vi "Test Lockin API.vi"() -> ()   [LabVIEW 2019]
uses:
  src/Instrument.Lockin/Instrument.Lockin.lvclass
  C:/Program Files (x86)/National Instruments/LabVIEW 2019/user.lib/LevyLab/Levylab Instruments/SMOs/Instrument/Instrument.lvclass
  src/Instrument.Lockinl.UI/Typedefs/Device Configuration--Cluster.ctl
  src/Lockin.DAQ/Typedefs/446xAO-enum.ctl
  src/Lockin.DAQ/Typedefs/446xAI-enum.ctl
  src/Lockin.DAQ/Typedefs/AI.coupling-enum.ctl
  <vilib>/addons/_JKI Toolkits/Caraya/classes/Test Suite/Define Test Suite (Default).vi
  <vilib>/addons/_JKI Toolkits/Caraya/classes/Test Suite/Test Suite.lvclass
  src/Lockin.DAQ/Lockin.DAQ.lvclass
  src/Instrument.Lockinl.UI/Instrument.Lockin.UI.lvclass
  <userlib>/LevyLab/Levylab Instruments/SMOs/Instrument/Instrument.lvclass
  C:/Program Files (x86)/National Instruments/LabVIEW 2019/vi.lib/JKI/JKI SMO/SMO/SMO.lvclass
panel:
  out "Instrument.Lockin out":refnum<class "Instrument.Lockin.lvclass">
  in  "Instrument.Lockin in":refnum<class "Instrument.Lockin.lvclass">
  # "NOTE:\nBefore running make sure that \"Same f\" = FALSE"
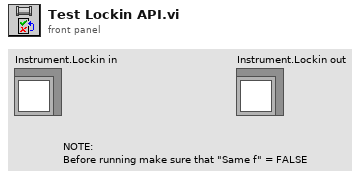
[diagram p1: front panel]
types:
  T1 = typedef "Instrument.Lockin.UI.lvclass/Device Configuration--Cluster.ctl" = cluster{"Device":string, "AO.Ch":string, "AO.Range":T2, "AI.Ch":string, "AI.Range":T3, "AI.Coupling":T4}
  T2 = typedef "Lockin.DAQ.lvclass/446xAO-enum.ctl" = enum16{"±0.1", "±1.0", "±10.0"}
  T3 = typedef "Lockin.DAQ.lvclass/446xAI-enum.ctl" = enum16{"±0.316", "±1.00", "±3.16", "±10.0", "±31.6", "±42.4"}
  T4 = typedef "Lockin.DAQ.lvclass/AI.coupling-enum.ctl" = u16
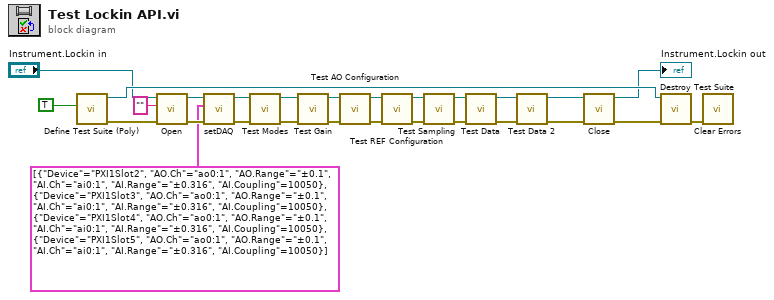
[diagram p0: block diagram]
diagram:
  n1 = call-poly <vilib>:"Define Test Suite (Poly).vi"("Interactive"=TRUE) -> ("error out"=w13:errorcluster, "Test Suite"=w22:refnum<class "Test Suite.lvclass">)  [unwired: 9 in]
  n2 = call <userlib>:"Open.vi"("error in (no error)"=w13, "address"="" ("Address"), "Instrument in"="Instrument.Lockin in") -> ("error out"=w9:errorcluster, "Instrument out"=w8:refnum<class "Instrument.Lockin.lvclass">)  [unwired: 7 in]
  n3 = call "setDAQ.vi"("error in (no error)"=w9, "setDAQ"=T1[] [{"Device"="PXI1Slot2", "AO.Ch"="ao0:1", "AO.Range"=enum."±0.1", "AI.Ch"="ai0:1", "AI.Range"=enum."±0.316", "AI.Coupling"=10050}, {"Device"="PXI1Slot3", "AO.Ch"="ao0:1", "AO.Range"=enum."±0.1", "AI.Ch"="ai0:1", "AI.Range"=enum."±0.316", "AI.Coupling"=10050}, {"Device"="PXI1Slot4", "AO.Ch"="ao0:1", "AO.Range"=enum."±0.1", "AI.Ch"="ai0:1", "AI.Range"=enum."±0.316", "AI.Coupling"=10050}, {"Device"="PXI1Slot5", "AO.Ch"="ao0:1", "AO.Range"=enum."±0.1", "AI.Ch"="ai0:1", "AI.Range"=enum."±0.316", "AI.Coupling"=10050}], "Instrument.Lockin in"=w8) -> ("error out"=w6:errorcluster, "Instrument.Lockin out"=w7:refnum<class "Instrument.Lockin.lvclass">)  [unwired: 7 in]
  n4 = call "Test Modes.vi"("error in (no error)"=w6, "Instrument.Lockin in"=w7) -> ("error out"=w21:errorcluster, "Instrument.Lockin out"=w27:refnum<class "Instrument.Lockin.lvclass">)  [unwired: 8 in]
  n5 = call "Test Gain.vi"("error in (no error)"=w21, "Instrument.Lockin in"=w27) -> ("error out"=w20:errorcluster, "Instrument.Lockin out"=w26:refnum<class "Instrument.Lockin.lvclass">)  [unwired: 8 in]
  n6 = call "Test AO Configuration.vi"("error in (no error)"=w20, "Instrument.Lockin in"=w26) -> ("error out"=w19:errorcluster, "Instrument.Lockin out"=w25:refnum<class "Instrument.Lockin.lvclass">)  [unwired: 8 in]
  n7 = call "Test REF Configuration.vi"("error in (no error)"=w19, "Instrument.Lockin in"=w25) -> ("error out"=w18:errorcluster, "Instrument.Lockin out"=w24:refnum<class "Instrument.Lockin.lvclass">)  [unwired: 8 in]
  n8 = call "Test Sampling.vi"("error in (no error)"=w18, "Instrument.Lockin in"=w24) -> ("error out"=w17:errorcluster, "Instrument.Lockin out"=w23:refnum<class "Instrument.Lockin.lvclass">)  [unwired: 8 in]
  n9 = call "Test Data.vi"("error in (no error)"=w17, "Instrument.Lockin in"=w23) -> ("error out"=w11:errorcluster, "Instrument.Lockin out"=w10:refnum<class "Instrument.Lockin.lvclass">)  [unwired: 8 in]
  n10 = call "Test Data 2.vi"("error in (no error)"=w11, "Instrument.Lockin in"=w10) -> ("error out"=w3:errorcluster, "Instrument.Lockin out"=w4:refnum<class "Instrument.Lockin.lvclass">)  [unwired: 8 in]
  n11 = call <userlib>:"Close.vi"("error in (no error)"=w3, "Instrument in"=w4) -> ("error out"=w1:errorcluster, "Instrument out"=→"Instrument.Lockin out":refnum<class "Instrument.Lockin.lvclass">)  [unwired: 8 in]
  n12 = call-dynamic "Destroy Test Suite.vi"("error in (no error)"=w1, "Test Suite in"=w22) -> ("error out"=w15:errorcluster)  [unwired: 8 in, 1 out]
  n13 = call <vilib>:"Clear Errors.vi"("error in (no error)"=w15) -> ()  [unwired: 5 in, 2 out]
